vi "CgtpReadVariableAsString.vi"(8 "progName":string, 9 "varName":string, 10 "Cgtp":refnum<k24>, 11 "error in":errorcluster) -> (2 "String Value":string, 3 "error out":errorcluster)   [LabVIEW 2011, in "UnderAutomation.Fanuc.lvlib"]
uses:
  UnderAutomation.Fanuc.lvlib
  C:/Users/fg/Documents/Fanuc.vi/LabVIEW_2024/UnderAutomation.Fanuc/lib/UnderAutomation.Fanuc.dll
  LabVIEW_2024/UnderAutomation.Fanuc/lib/UnderAutomation.Fanuc.dll
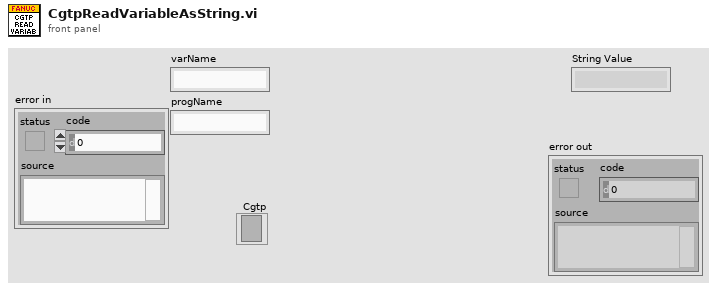
[diagram p1: front panel]
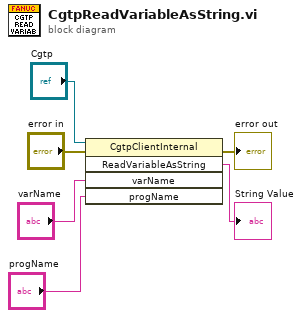
[diagram p0: block diagram]
diagram:
  n1 = invoke class="CgtpClientInternal" method="ReadVariableAsString"(reference="Cgtp", error in="error in", "varName"="varName", "progName"="progName") -> (error out=→"error out":errorcluster, "ReadVariableAsString"=→"String Value":string)  [unwired: 1 in, 3 out]
